vi "Set Description.vi"(8 "error in":errorcluster, 10 "description":string, 11 "Ballard ARINC 429 custom device in":T1 format="%.0x") -> (0 "error out":errorcluster, 3 "Ballard ARINC 429 custom device out":T1 format="%.0x")   [LabVIEW 2020, in "AIM ARINC 429 Scripting.lvlib"]
doc: "Writes the <b>description</b> field for the input <b>Ballard ARINC 429 custom device</b>."
uses:
  AIM ARINC 429 Scripting.lvlib
  <vilib>/NI VeriStand/Custom Device API/Custom Device Item Ref.ctl
  <vilib>/NI VeriStand/Custom Device API/Custom Device API.lvlib
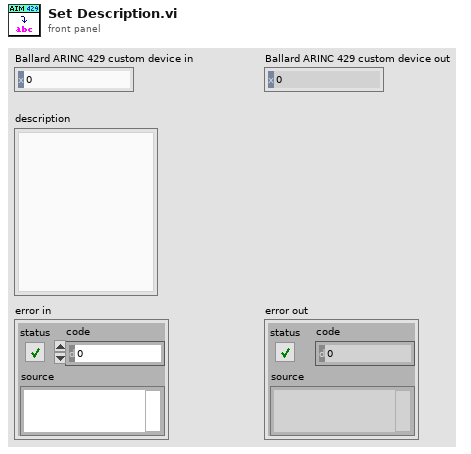
[diagram p1: front panel]
types:
  T1 = typedef "Custom Device API.lvlib/Custom Device Item Ref.ctl" = u64
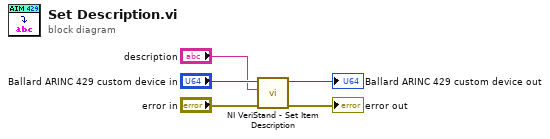
[diagram p0: block diagram]
diagram:
  n1 = call <vilib>:"NI VeriStand - Set Item Description.vi"("error in (no error)"="error in", "Description"="description", "Item Ref in"="Ballard ARINC 429 custom device in") -> ("error out"=→"error out":errorcluster, "Item Ref out"=→"Ballard ARINC 429 custom device out":T1)  [unwired: 6 in, 1 out]
